vi "Zarlink Telemetry.vi"(8 "error in (no error)":errorcluster, 10 "Input":T3={"Command"=enum."Get xPG Status", "Function"=enum."Transceive (DN -> UP)", "MICS_ID"=0, "EXID"=16773121, "Use Local"=FALSE, "Transceive Delay mS"=200.0, "CP_DATA IN"=[], "Parameters"=""} {"Transceive Delay mS" min=0.0 max=10000.0 step=1.0; "EXID" step=1 format="%.0x"; "MICS_ID" step=1 format="%04x"}, 11 "MICS Dongle Address":refnum<visa-resource-name>="COM5") -> (0 "error out":errorcluster, 1 "Status Flags":T1, 2 "Output":T4)   [LabVIEW 2020]
uses:
  Typedef Command List.ctl
  <vilib>/Instr/_visa.llb/VISA Configure Serial Port (Instr).vi
  MICS_ID Global.vi
  MICS_Channel Global.vi
  MICS Parameters Global.vi
  <vilib>/Utility/file.llb/Write To Spreadsheet File (string).vi
panel:
  out "MICS ID":u32 format="%.0x"
  in  "Use MICS Dongle":bool=TRUE
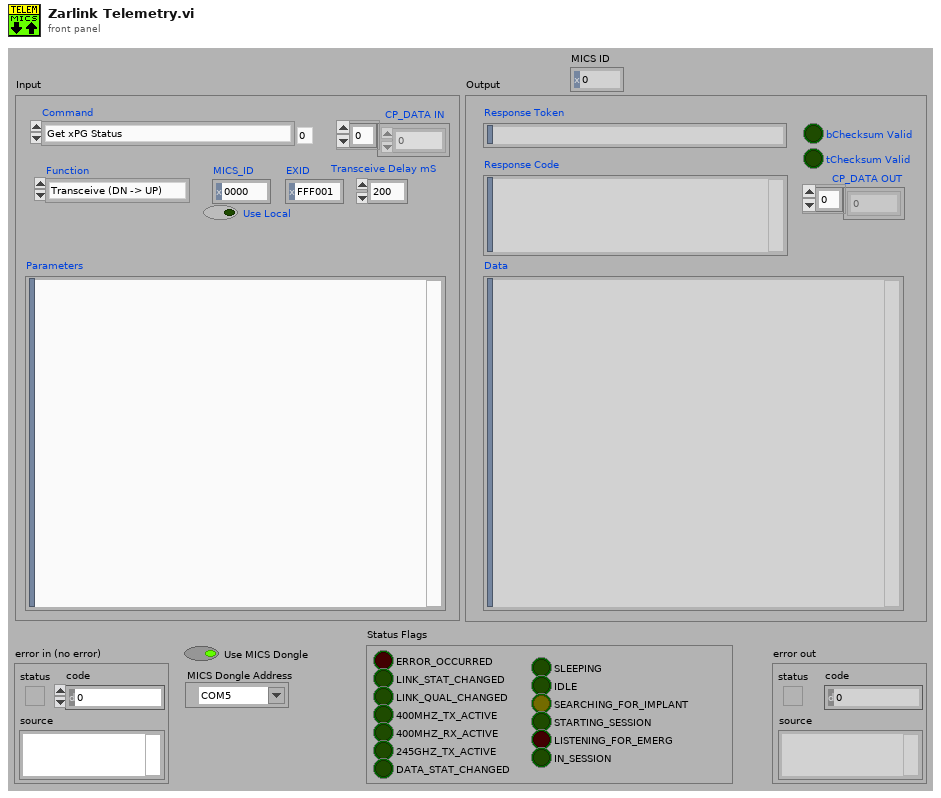
[diagram p1: front panel]
types:
  T1 = cluster{"ERROR_OCCURRED":bool, "LINK_STAT_CHANGED":bool, "LINK_QUAL_CHANGED":bool, "400MHZ_TX_ACTIVE":bool, "400MHZ_RX_ACTIVE":bool, "245GHZ_TX_ACTIVE":bool, "DATA_STAT_CHANGED":bool, "SLEEPING":bool, "IDLE":bool, "SEARCHING_FOR_IMPLANT":bool, "STARTING_SESSION":bool, "LISTENING_FOR_EMERG":bool, "IN_SESSION":bool}
  T2 = typedef "Typedef Command List.ctl" = enum16{"Get xPG Status", "xPG Stimulation", "Select Program", "Increment Program Amplitude", "Decrement Program Amplitude", "Get PoP Constants", "Get PPC Constants", "Get Program Names", "Set Pulse Amplitude", "Increment Pulse Amplitude", "Decrement Pulse Amplitude", "Get Pulse Widths", "Set Pulse Widths", "Increment Pulse Width", "Decrement Pulse Width", "Get Program Frequency", "Set Program Frequency", "Increment Program Frequency", "Decrement Program Frequency", "Inject Event", "Charging Control", "Get xPG Identity", "Set xPG Identity", "Restore Program Defaults", "Get Program Definition", "Set Program Definition", "Get Program Constants", "Set Program Constants", "Get Configurable Device Parameters", "Set Configurable Device Parameters", "Get Pulse Constants", "Set Pulse Constants", "Get Lead Limits", "Set Lead Limits", "Get Channel Calibrations", "Set Channel Calibrations", "<reserved 2>", "<reserved 3>", "<reserved 4>", "<reserved 5>", "<reserved 6>", "<reserved 7>", "Get Stim Asic HV Calibrations", "Set Stim Asic HV Calibrations", "<reserved 8>", "<reserved 9>", "Get CP Data", "Set CP Data", "Clear Log", "Read Log", "Append Log", "Get Patient Program Runtime", "Set Patient Program Runtime", "Impedance Measurement", "Enter Storage Mode", "Echo Short", "Echo Long", "Get General Calibration", "Set General Calibration", "Get Trim List", "Set Trim List", "Get Counter", "Set Counter", "Get Test Stimulation", "Set Test Stimulation", "Get Titration Stimulation", "Set Titration Stimulation", "Get Ramp Time", "Set Ramp Time", "Get VBAT", "Set Software Description Block", "Get Software Description Block", "Write Memory", "Read Memory", "Reset xPG", "Erase Flash Block", "Write Vectors", "Read Vectors", "Diagnostic Data", "Set Background Impedance", "Get Background Impedence ", "Set Test Waveform", "Calibrate Channel", "Get Log Range", "Reserved 0x55", "Reserved 0x56", "MICS Options", "Pair PPC", "Pair POP", "Stop Bootloader", "Tune MICS", "MICS Diagnostics", "Undefined"}
  T3 = cluster{"Command":T2, "Function":enum16{"Open Session", "Close Session", "Downlink Only", "Uplink Only", "Transceive (DN -> UP)"}, "MICS_ID":u32, "EXID":u32, "Use Local":bool, "Transceive Delay mS":dbl, "CP_DATA IN":u8[], "Parameters":string}
  T4 = cluster{"Response Token":string, "Response Code":string, "bChecksum Valid":bool, "tChecksum Valid":bool, "CP_DATA OUT":u8[], "Data":string}
  T5 = cluster{"ConfigFlags":u8, "ImplantID":u32, "CompanyID":u8, "Normal_Comm":cluster{"RF_Channel":u8, "UserData":u8, "TX_Mod":u8, "RX_Mod":u8, "RX_BlockSize":u8, "BlockPerPack":u8, "TX_BlockSize":u8}, "Emerg_Comm":cluster{"RF_Channel":u8, "UserData":u8, "TX_Mod":u8, "RX_Mod":u8, "TX_BlockSize":u8, "BlockPerPack":u8, "RX_BlockSize":u8}, "ImplantRev":u8, "245TX_PowerCal":i8, "245TX_Power":i8, "CCA_RSSI_Thresholds":cluster{"ch0":u16, "ch1":u16, "ch2":u16, "ch3":u16, "ch4":u16, "ch5":u16, "ch6":u16, "ch7":u16, "ch8":u16, "ch9":u16}}
  T6 = enum16{"Open Session", "Close Session", "Downlink Only", "Uplink Only", "Transceive (DN -> UP)"}
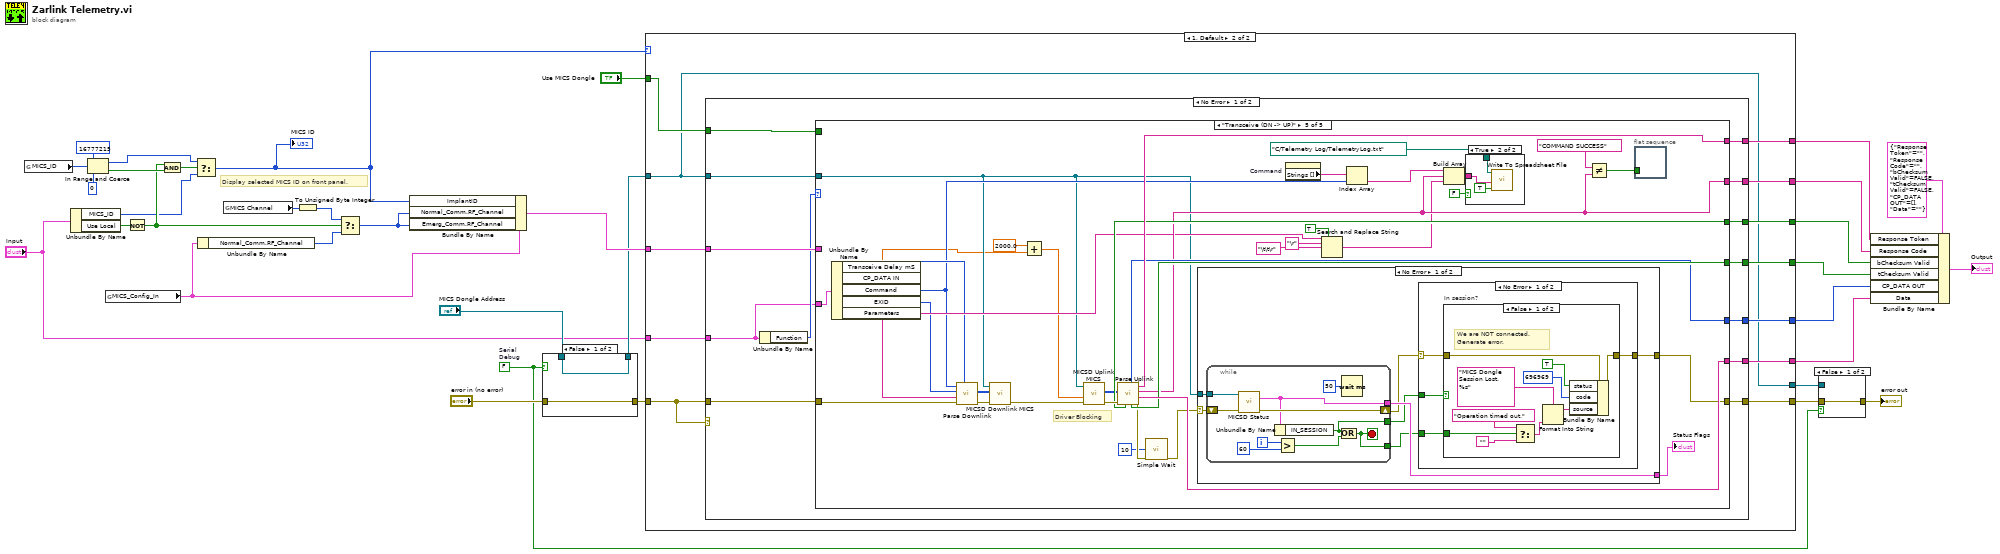
[diagram p0: block diagram]
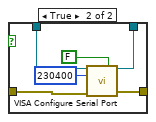
[diagram p2: hidden frame]
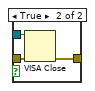
[diagram p3: hidden frame]
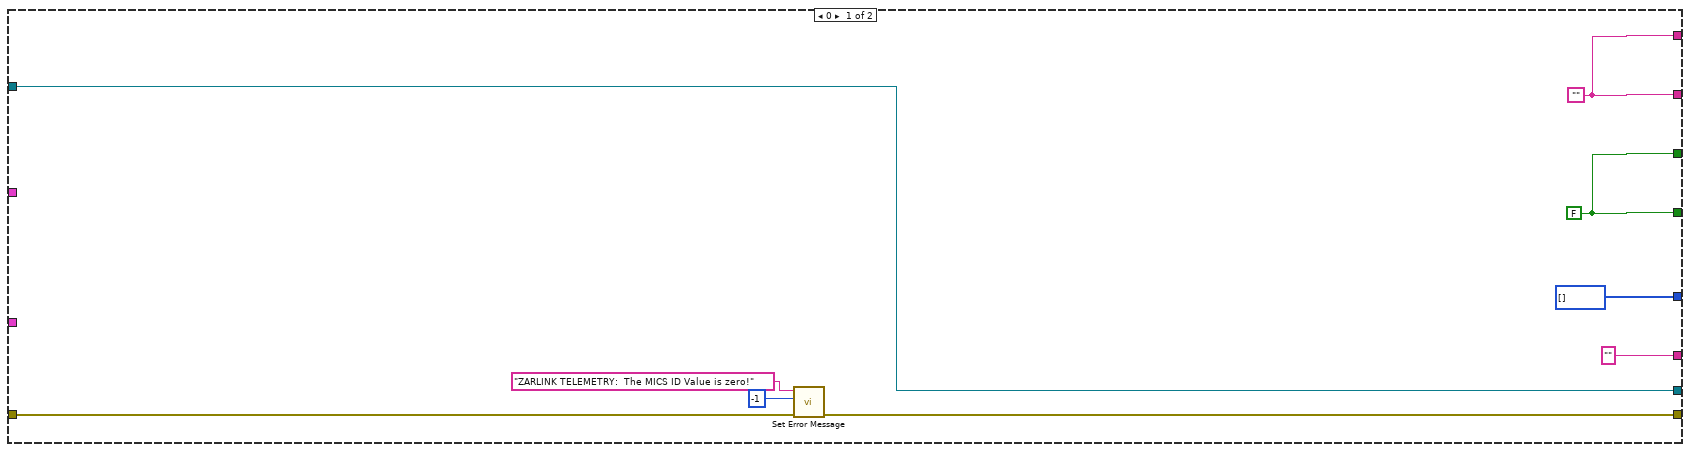
[diagram p4: hidden frame]
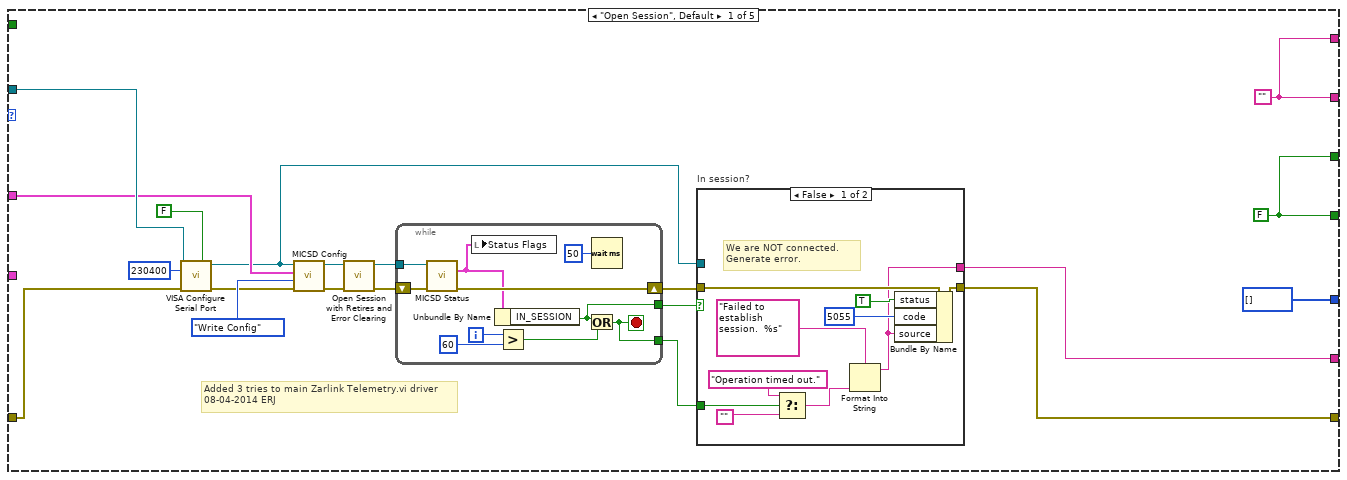
[diagram p5: hidden frame]
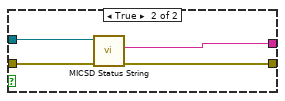
[diagram p6: hidden frame]
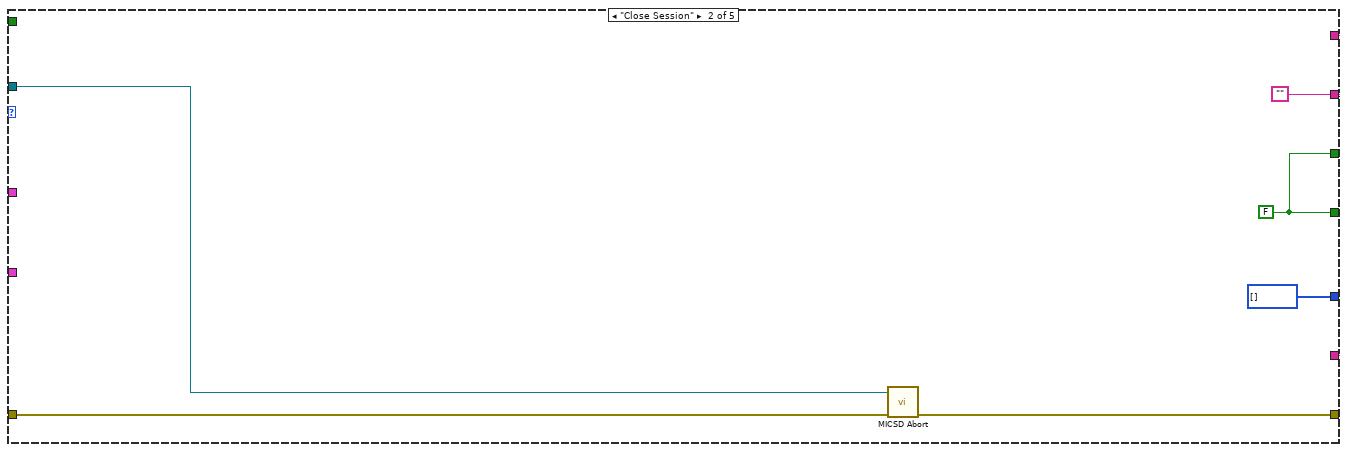
[diagram p7: hidden frame]
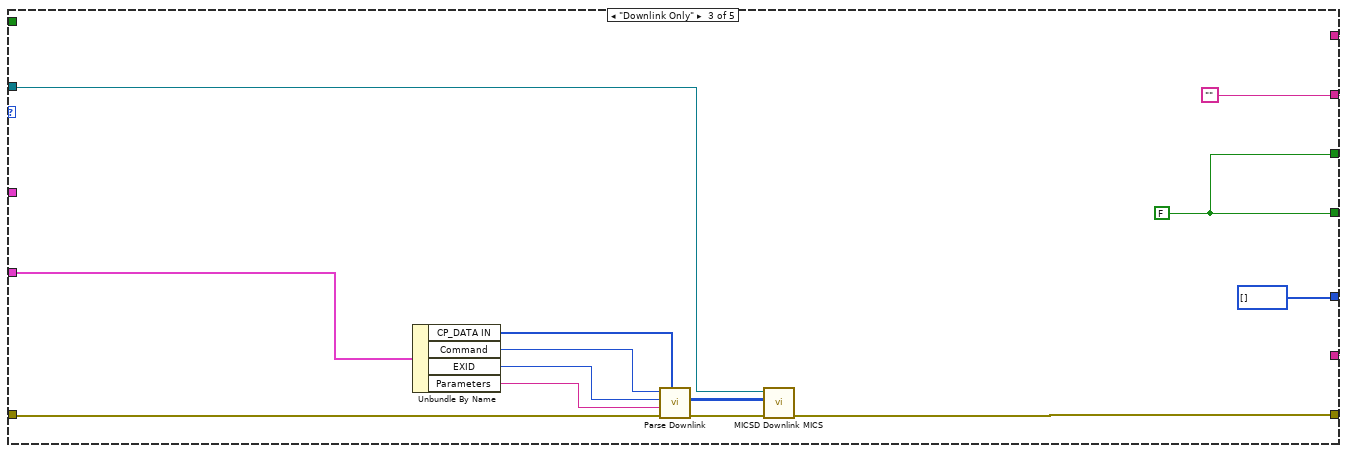
[diagram p8: hidden frame]
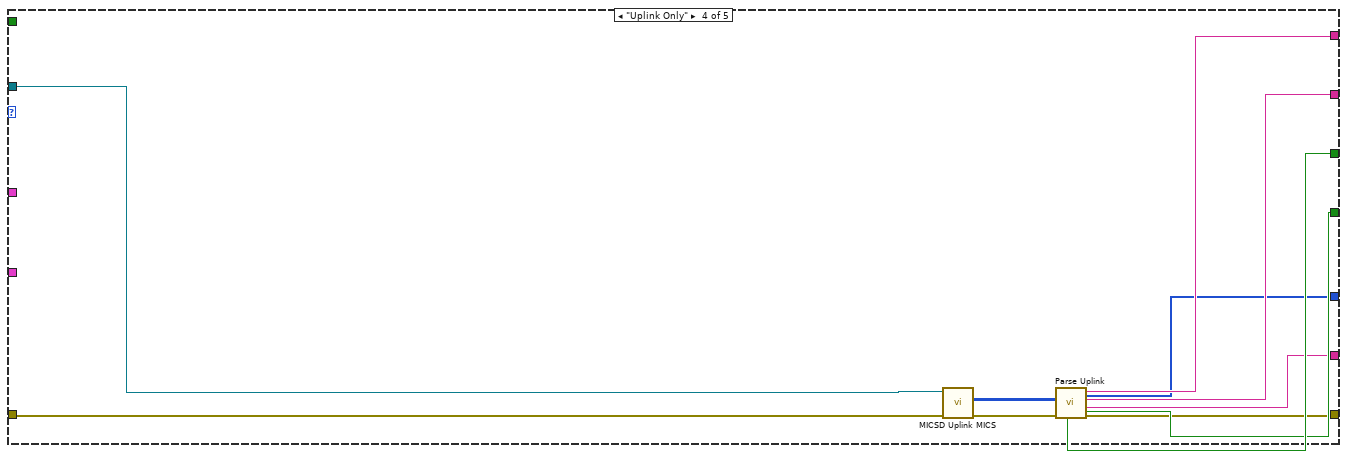
[diagram p9: hidden frame]
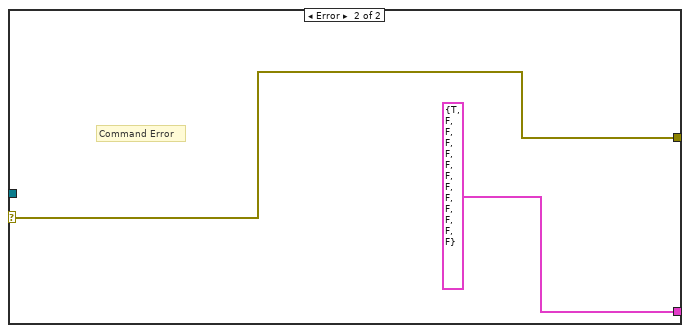
[diagram p12: hidden frame]
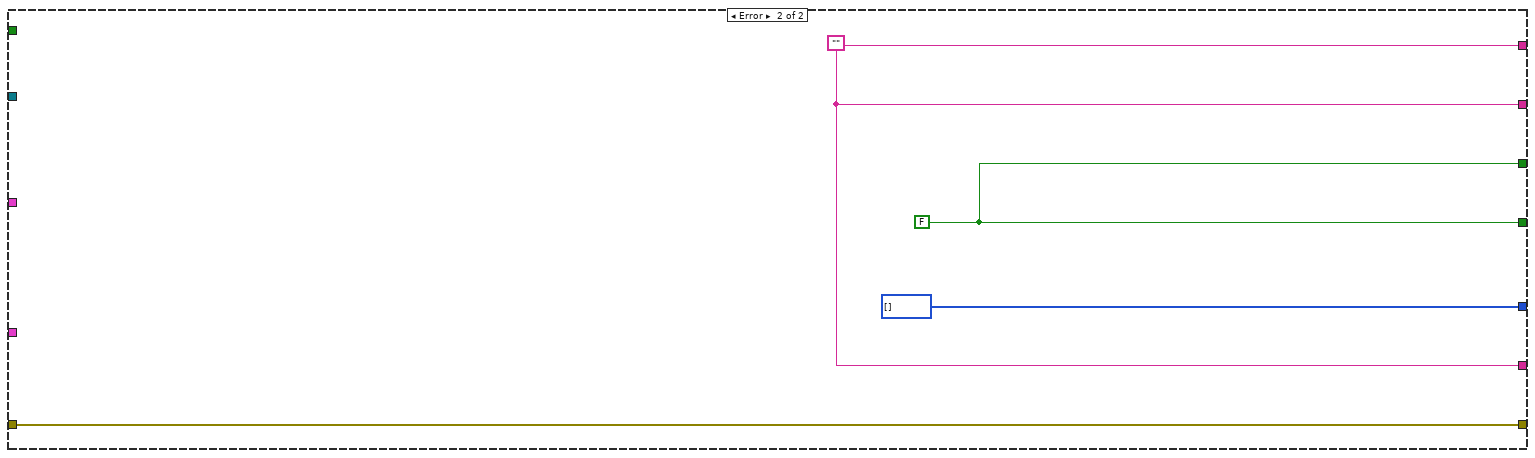
[diagram p14: hidden frame]
diagram:
  w6 = FALSE  # Serial  Debug
  # "Display selected MICS ID on front panel."
  n1 = global read "MICS_ID Global.vi" "MICS_ID"() -> (w34:u32)
  n2 = Unbundle By Name("Input") -> ("MICS_ID"=w14:u32, "Use Local"=w15:bool)
  n3 = In Range and Coerce(upper limit=u32 16777215, x=w34, lower limit=u32 0) -> (coerced(x)=w29:u32, In Range?=w31:bool)
  n4 = global read "MICS Parameters Global.vi" "MICS_Config_In"() -> (w3:T5)
  n5 = Not(x=w15) -> (.not. x?=w27:bool)
  n6 = And(x=w27, y=w31) -> (x .and. y?=w30:bool)
  n7 = Select(t=w29, s=w30, f=w14) -> (s? t:f=w5:u32)
  "MICS ID" <- w5
  n8 = Unbundle By Name(w3) -> ("Normal_Comm.RF_Channel"=w2:u8)
  n9 = global read "MICS_Channel Global.vi" "MICS Channel"() -> (w28:u16)
  n10 = To Unsigned Byte Integer(number=w28) -> (unsigned 8bit integer=w1:u8)
  n11 = Select(t=w1, s=w27, f=w2) -> (s? t:f=w24:u8)
  n12 = Bundle By Name(cluster=w3, "ImplantID"=w5, "Normal_Comm.RF_Channel"=w24, "Emerg_Comm.RF_Channel"=w24) -> (w25:T5)
  n13 = case shown="False" w6 {
    tunnel: [w36 w40] -> w13
    tunnel: "error in (no error)" -> [w36 w39]
    tunnel: "MICS Dongle Address" -> [w35 w38]
    tunnel: [w35 w37] -> w10
    frame False {
    }
    frame True {
      n14 = call-poly "VISA Configure Serial Port"("VISA resource name"=w38, "Enable Termination\nChar (T)"=FALSE ("Enable Termination\nChar (T)"), "baud rate (9600)"=u32 230400, "error in (no error)"=w39) -> ("VISA resource name out"=w37:refnum<visa-resource-name>, "error out"=w40:errorcluster)  [unwired: 10 in]
    }
  }
  n15 = case shown="1, Default" w5 {
    tunnel: [w45 w63] -> w9
    tunnel: w13 -> [w46 w62]
    tunnel: [w49 w61] -> w21
    tunnel: [w49 w60] -> w20
    tunnel: [w50 w59] -> w18
    tunnel: [w50 w58] -> w17
    tunnel: [u8[] [] ("CP_DATA OUT") w57] -> w16
    tunnel: ["" ("Data") w56] -> w19
    tunnel: w10 -> [w47 w52]
    tunnel: "Use MICS Dongle" -> [_ w55]
    tunnel: w25 -> [_ w54]
    tunnel: "Input" -> [_ w53]
    tunnel: [w47 w52] -> w7
    frame 0 {
      w49 = ""
      w50 = FALSE
      n16 = call "Set Error Message.vi"("error in"=w46, "code (-1)"=-1 ("code"), "message"="ZARLINK TELEMETRY:  The MICS ID Value is zero!") -> ("error out"=w45:errorcluster)  [unwired: 5 in]
    }
    frame 1, Default {
      n17 = case shown="No Error" w62 {
        tunnel: w62 -> [w76 w229]
        tunnel: [w75 w229] -> w63
        tunnel: [w69 w226] -> w61
        tunnel: [w70 w226] -> w60
        tunnel: [w71 w228] -> w59
        tunnel: [w72 w228] -> w58
        tunnel: [w73 u8[] [] ("CP_DATA OUT")] -> w57
        tunnel: [w74 w226] -> w56
        tunnel: w52 -> [w68 _]
        tunnel: w55 -> [w67 _]
        tunnel: w54 -> [w66 _]
        tunnel: w53 -> [w64 _]
        frame No Error {
          n18 = Unbundle By Name(w64) -> ("Function"=w65:T6)
          n19 = case shown="\"Transceive (DN -> UP)\"" w65 {
            tunnel: w76 -> [w91 w124 w137 w141 w186]
            tunnel: [w92 w123 w133 w142 w156] -> w75
            tunnel: [w93 w122 w134 w143 w184] -> w74
            tunnel: [u8[] [] ("CP_DATA OUT") u8[] [] ("CP_DATA OUT") u8[] [] ("CP_DATA OUT") w144 w180] -> w73
            tunnel: [w96 w125 w136 w145 w181] -> w72
            tunnel: [w96 w125 w136 w146 w182] -> w71
            tunnel: [w95 w122 w134 w147 w174] -> w70
            tunnel: [w95 w122 w134 w148 w183] -> w69
            tunnel: w68 -> [w90 w121 w132 w140 w157]
            tunnel: w67 -> [_ _ _ _ _]
            tunnel: w66 -> [w89 _ _ _ _]
            tunnel: w64 -> [_ _ w131 _ w166]
            frame "Open Session", Default {
              w95 = ""
              w96 = FALSE
              # "Added 3 tries to main Zarlink Telemetry.vi driver\n08-04-2014 ERJ"
              n20 = call-poly "VISA Configure Serial Port"("VISA resource name"=w90, "Enable Termination\nChar (T)"=FALSE ("Enable Termination\nChar (T)"), "baud rate (9600)"=u32 230400, "error in (no error)"=w91) -> ("VISA resource name out"=w81:refnum<visa-resource-name>, "error out"=w82:errorcluster)  [unwired: 10 in]
              n21 = call "MICSD Config.vi"("error in (no error)"=w82, "Function"=enum16{"Write Config", "Read Config"}."Write Config", "MICS_Config_In"=w89, "VISA Resource Name"=w81) -> ("error out"=w78:errorcluster, "dup VISA Resource Name"=w80:refnum<visa-resource-name>)  [unwired: 5 in, 1 out]
              n22 = call "Open Session with Retires and Error Clearing.vi"("error in"=w78, "VISA Resource Name"=w80) -> ("error out"=w77:errorcluster, "dup VISA Resource Name"=w79:refnum<visa-resource-name>)  [unwired: 6 in, 2 out]
              n23 = while {
                tunnel: w79 -> [w119]
                shift-right: [w118] -> w86
                shift-left: w77 -> [w120]
                tunnel: [w113] -> w87
                tunnel: [w112] -> w85
                i -> [w115]
                stop <- w112 stop-if-true
                n24 = call "MICSD Status.vi"("VISA Resource Name"=w119, "error in (no error)"=w120) -> ("Status Flags"=w111:T1, "error out"=w118:errorcluster)  [unwired: 7 in, 5 out]
                n25 = local write "Status Flags"(w111) -> ()
                n26 = Unbundle By Name(w111) -> ("IN_SESSION"=w113:bool)
                n27 = Greater?(x=w115, y=60) -> (0:w116:bool)
                n28 = Or(x=w113, y=w116) -> (x .or. y?=w112:bool)
                n29 = Wait (ms)(milliseconds to wait=u32 50) -> ()  [unwired: 1 out]
              }
              n30 = case "In session?" shown="False" w87 {
                tunnel: w86 -> [w106 w110]
                tunnel: [w100 w109] -> w92
                tunnel: w85 -> [w104 _]
                tunnel: [w97 w107] -> w93
                tunnel: w81 -> [_ w108]
                frame False {
                  # "We are NOT connected. Generate error."
                  n31 = Select(t="Operation timed out." ("format string"), s=w104, f="") -> (s? t:f=w99:string)
                  n32 = Format Into String(format string="Failed to establish session.  %s", w99) -> (resulting string=w97:string)  [unwired: 2 in, 1 out]
                  n33 = Bundle By Name(cluster=w106, "status"=TRUE, "code"=5055, "source"=w97) -> (w100:errorcluster)
                }
                frame True {
                  n34 = call "MICSD Status String.vi"("error in (no error)"=w110, "VISA Resource Name"=w108) -> ("error out"=w109:errorcluster, "Response"=w107:string)  [unwired: 7 in, 1 out]
                }
              }
            }
            frame "Close Session" {
              w122 = ""
              w125 = FALSE
              n35 = call "MICSD Abort.vi"("error in (no error)"=w124, "VISA Resource Name"=w121) -> ("error out"=w123:errorcluster)  [unwired: 8 in, 1 out]
            }
            frame "Downlink Only" {
              w134 = ""
              w136 = FALSE
              n36 = Unbundle By Name(w131) -> ("CP_DATA IN"=w130:u8[], "Command"=w129:T2, "EXID"=w128:u32, "Parameters"=w127:string)
              n37 = call "Parse Downlink.vi"("CP_DATA IN"=w130, "error in (no error)"=w137, "Parameters"=w127, "EXID"=w128, "Command"=w129) -> ("error out"=w139:errorcluster, "Downlink"=w138:u8[][])  [unwired: 5 in]
              n38 = call "MICSD Downlink MICS.vi"("Error In"=w139, "Downlink"=w138, "VISA Resource Name"=w132) -> ("Error Out"=w133:errorcluster)  [unwired: 7 in, 1 out]
            }
            frame "Uplink Only" {
              n39 = call "MICSD Uplink MICS.vi"("Error In"=w141, "VISA Resource Name"=w140) -> ("Error Out"=w150:errorcluster, "Uplink"=w149:u8[][])  [unwired: 7 in, 1 out]
              n40 = call "Parse Uplink.vi"("error in (no error)"=w150, "Uplink"=w149) -> ("error out"=w142:errorcluster, "Data"=w143:string, "Response Code"=w147:string, "Response Token"=w148:string, "tChecksum Valid"=w145:bool, "CP_DATA"=w144:u8[], "bChecksum Valid"=w146:bool)  [unwired: 3 in]
            }
            frame "Transceive (DN -> UP)" {
              # "Driver Blocking"
              n41 = Unbundle By Name(w166) -> ("Transceive Delay mS"=w152:dbl, "CP_DATA IN"=w164:u8[], "Command"=w162:T2, "EXID"=w163:u32, "Parameters"=w165:string)
              n42 = call "Parse Downlink.vi"("CP_DATA IN"=w164, "error in (no error)"=w186, "Parameters"=w165, "EXID"=w163, "Command"=w162) -> ("error out"=w187:errorcluster, "Downlink"=w161:u8[][])  [unwired: 5 in]
              n43 = call "MICSD Downlink MICS.vi"("Error In"=w187, "Downlink"=w161, "VISA Resource Name"=w157) -> ("Error Out"=w154:errorcluster)  [unwired: 7 in, 1 out]
              n44 = Add(x=2000.0, y=w152) -> (x+y=w151:dbl)
              n45 = call "MICSD Uplink MICS.vi"("Error In"=w154, "Timeout(mS)"=w151, "VISA Resource Name"=w157) -> ("Error Out"=w185:errorcluster, "Uplink"=w179:u8[][])  [unwired: 6 in, 1 out]
              n46 = call "Parse Uplink.vi"("error in (no error)"=w185, "Uplink"=w179) -> ("error out"=w160:errorcluster, "Data"=w184:string, "Response Code"=w174:string, "Response Token"=w183:string, "tChecksum Valid"=w181:bool, "CP_DATA"=w180:u8[], "bChecksum Valid"=w182:bool)  [unwired: 3 in]
              n47 = call "Simple Wait.vi"("mS"=u32 10, "error in"=w160) -> ("error out"=w155:errorcluster)  [unwired: 12 in, 1 out]
              n48 = case shown="No Error" w155 {
                selector: w155 -> [w189 w221]
                tunnel: [w194 T1 {"ERROR_OCCURRED"=TRUE, "LINK_STAT_CHANGED"=FALSE, "LINK_QUAL_CHANGED"=FALSE, "400MHZ_TX_ACTIVE"=FALSE, "400MHZ_RX_ACTIVE"=FALSE, "245GHZ_TX_ACTIVE"=FALSE, "DATA_STAT_CHANGED"=FALSE, "SLEEPING"=FALSE, "IDLE"=FALSE, "SEARCHING_FOR_IMPLANT"=FALSE, "STARTING_SESSION"=FALSE, "LISTENING_FOR_EMERG"=FALSE, "IN_SESSION"=FALSE} ("Status Flags")] -> w158
                tunnel: w157 -> [w193 _]
                tunnel: [w192 w221] -> w156
                frame No Error {
                  n49 = while {
                    tunnel: w193 -> [w219]
                    shift-right: [w218] -> w188
                    shift-left: w189 -> [w220]
                    tunnel: [w213] -> w191
                    tunnel: [w212] -> w190
                    tunnel: [w211] -> w194
                    i -> [w215]
                    stop <- w212 stop-if-true
                    n50 = call "MICSD Status.vi"("VISA Resource Name"=w219, "error in (no error)"=w220) -> ("Status Flags"=w211:T1, "error out"=w218:errorcluster)  [unwired: 7 in, 5 out]
                    n51 = Unbundle By Name(w211) -> ("IN_SESSION"=w213:bool)
                    n52 = Greater?(x=w215, y=60) -> (0:w216:bool)
                    n53 = Or(x=w213, y=w216) -> (x .or. y?=w212:bool)
                    n54 = Wait (ms)(milliseconds to wait=u32 50) -> ()  [unwired: 1 out]
                  }
                  n55 = case shown="No Error" w188 {
                    selector: w188 -> [w195 w210]
                    tunnel: [w198 w210] -> w192
                    tunnel: w191 -> [w197 _]
                    tunnel: w190 -> [w196 _]
                    frame No Error {
                      n56 = case "In session?" shown="False" w197 {
                        tunnel: w195 -> [w199 w209]
                        tunnel: [w203 w209] -> w198
                        tunnel: w196 -> [w207 _]
                        frame False {
                          # "We are NOT connected. Generate error."
                          n57 = Select(t="Operation timed out." ("format string"), s=w207, f="") -> (s? t:f=w202:string)
                          n58 = Format Into String(format string="MICS Dongle Session Lost.  %s", w202) -> (resulting string=w200:string)  [unwired: 2 in, 1 out]
                          n59 = Bundle By Name(cluster=w199, "status"=TRUE, "code"=696969, "source"=w200) -> (w203:errorcluster)
                        }
                        frame True {
                        }
                      }
                    }
                    frame Error {
                      # "Pass the error if it occurs because\nof inability to get Base Station Status."
                    }
                  }
                }
                frame Error {
                  # "Command Error"
                }
              }
              "Status Flags" <- w158
              n60 = property on="Command" class="Enum (strict)"() -> ("Strings []"=w176:string[])  [unwired: 2 in, 2 out]
              n61 = Search and Replace String(replace all?=TRUE ("replace all? (F)"), input string=w165, search string="\r", replace string="\t\t\r" ("search string")) -> (result string=w171:string)  [unwired: 4 in, 3 out]
              n62 = Index Array(array=w176, index=w162) -> (element=w175:string)
              n63 = Build Array(w175, w174, w171) -> (w172:string[])
              n64 = case shown="True" FALSE {
                tunnel: path "C:/Telemetry Log/TelemetryLog.txt" ("file (use dialog)") -> [_ w225]
                tunnel: w172 -> [_ w224]
                frame False {
                }
                frame True {
                  n65 = call-poly <vilib>:"Write To Spreadsheet File.vi"("append to file? (new file:F)"=TRUE, "1D data"=w224, "file path (dialog if empty)"=w225) -> ()  [unwired: 5 in, 1 out]
                }
              }
              n66 = Not Equal?(x="COMMAND SUCCESS", y=w174) -> (x != y?=w177:bool)
              n67 = flat-sequence {
                tunnel: w177 -> [_]
                frame #0 {
                }
              }
            }
          }
        }
        frame Error {
          w226 = ""
          w228 = FALSE
        }
      }
    }
  }
  n68 = case shown="False" w6 {
    tunnel: w9 -> [w230 w233]
    tunnel: [w230 w232] -> w8
    tunnel: w7 -> [_ w231]
    frame False {
    }
    frame True {
      n69 = VISA Close(VISA resource name=w231, error in (no error)=w233) -> (error out=w232:errorcluster)
    }
  }
  "error out" <- w8
  n70 = Bundle By Name(cluster=T4 {"Response Token"="", "Response Code"="", "bChecksum Valid"=FALSE, "tChecksum Valid"=FALSE, "CP_DATA OUT"=[], "Data"=""} ("Output"), "Response Token"=w21, "Response Code"=w20, "bChecksum Valid"=w18, "tChecksum Valid"=w17, "CP_DATA OUT"=w16, "Data"=w19) -> (→"Output":T4)
